vi "Msg.vi"(7 "jettl in":refnum<class "jettl.lvclass">, 11 "Create Event Msg Strategy in":refnum<class "Create Event Msg Strategy.lvclass">) -> (5 "jettl out":refnum<class "jettl.lvclass">)   [LabVIEW 2021, in "jettl Msg Create Event.lvlib" / "Create Event Msg Strategy.lvclass"]
uses:
  Create Event Msg Strategy.lvclass
  Create Event Msg Strategy.lvclass/Create Event Msg Strategy.ctl
  Create Event/Create Event.lvclass
  jettl/jettl/jettl.lvclass
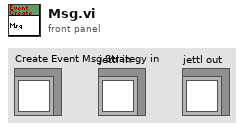
[diagram p1: front panel]
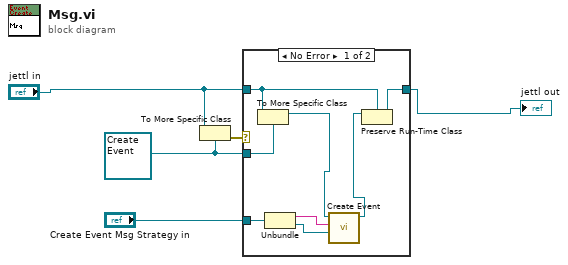
[diagram p0: block diagram]
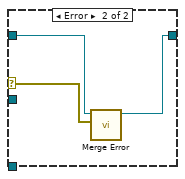
[diagram p2: hidden frame]
diagram:
  w2 = refnum<class "Create Event.lvclass"> refnum ("Event Create.lvlib:Event Create.lvclass")
  n1 = To More Specific Class(target class=w2, reference="jettl in") -> (error out=w5:errorcluster)  [unwired: 1 in, 1 out]
  n2 = case shown="No Error" w5 {
    selector: w5 -> [_ w16]
    tunnel: [w11 w14] -> w1
    tunnel: "jettl in" -> [w12 w15]
    tunnel: w2 -> [w13 _]
    tunnel: "Create Event Msg Strategy in" -> [w8 _]
    frame No Error {
      n3 = To More Specific Class(target class=w13, reference=w12) -> (specific class reference=w9:refnum<class "Create Event.lvclass">)  [unwired: 1 in, 1 out]
      n4 = Unbundle(w8) -> (w7:string, w6:refnum<class "Event jettl.lvclass">)
      n5 = call-dynamic "Create Event.vi"("Event jettl"=w6, "Alias"=w7, "Create Event in"=w9) -> ("Create Event out"=w10:refnum<class "Create Event.lvclass">)  [unwired: 8 in]
      n6 = Preserve Run-Time Class(object in=w10, 2:w12) -> (object out=w11:refnum<class "jettl.lvclass">)  [unwired: 1 in, 1 out]
    }
    frame Error {
      n7 = call-dynamic "Merge Error.vi"("Error"=w16, "Merge Error in"=w15) -> ("Merge Error out"=w14:refnum<class "jettl.lvclass">)  [unwired: 9 in]
    }
  }
  "jettl out" <- w1
